vi "Test_RequestInvalidTopic_ReturnError.vi"(8 "error in (no error)":errorcluster, 11 "TestCase in":refnum<class "TestTopicLookupTable.lvclass">) -> (0 "error out":errorcluster, 3 "TestCase out":refnum<class "TestTopicLookupTable.lvclass">)   [LabVIEW 2017, in "TestTopicLookupTable.lvclass"]
uses:
  TestTopicLookupTable.lvclass
  Source/Mediator/TopicLookupTable/TopicLookupTable.lvclass/TopicLookupTable.ctl
  gpm_packages/@cs/variant/Source/Format Type String.vi
  <vilib>/ActorFramework/Message Enqueuer/Message Enqueuer.lvclass
  Source/Mediator/TopicLookupTable/TopicLookupTable.lvclass
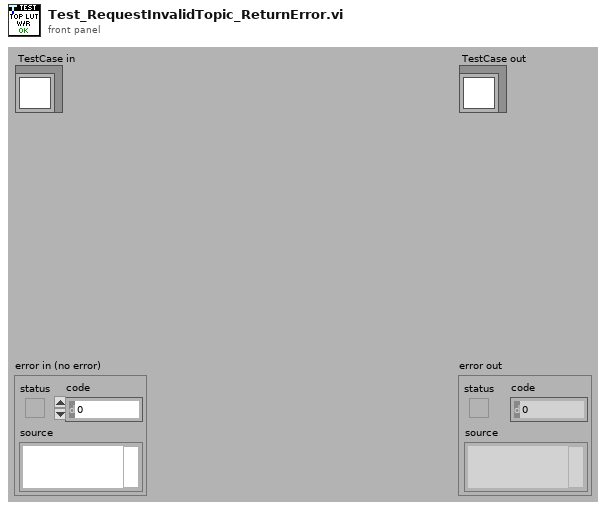
[diagram p1: front panel]
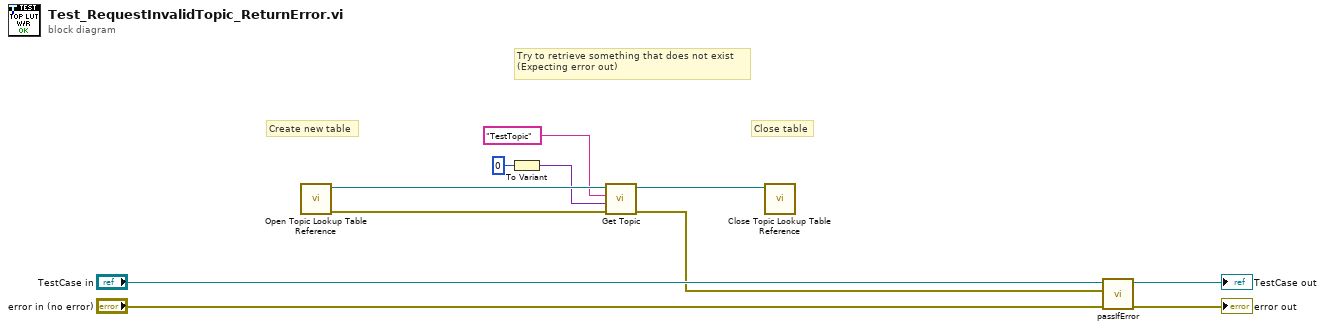
[diagram p0: block diagram]
diagram:
  # "Close table"
  # "Create new table"
  # "Try to retrieve something that does not exist\n(Expecting error out)"
  n1 = call "Open Topic Lookup Table Reference.vi"() -> ("error out"=w6:errorcluster, "TopicLookupTable Reference"=w7:refnum<data-value>)  [unwired: 10 in]
  n2 = To Variant(anything=0) -> (Variant=w1:variant)
  n3 = call "Get Topic.vi"("error in (no error)"=w6, "Topic Type"=w1, "Topic Name"="TestTopic", "TopicLookupTable"=w7) -> ("error out"=w3:errorcluster, "TopicLookupTable"=w5:refnum<data-value>)  [unwired: 5 in, 1 out]
  n4 = call "Close Topic Lookup Table Reference.vi"("TopicLookupTable"=w5) -> ()  [unwired: 10 in, 1 out]
  n5 = call-dynamic "passIfError.vi"("error in (no error)"="error in (no error)", "error"=w3, "TestCase in"="TestCase in") -> ("error out"=→"error out":errorcluster, "TestCase out"=→"TestCase out":refnum<class "TestTopicLookupTable.lvclass">)  [unwired: 7 in]
